vi "Calculate_TargetOffset_Method1.vi"(9 "distance":dbl, 10 "skew":dbl, 11 "depth":dbl) -> (1 "max possible":dbl, 3 "target offset":dbl)   [LabVIEW 2019]
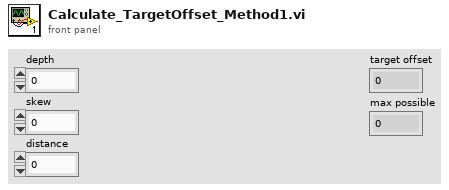
[diagram p1: front panel]
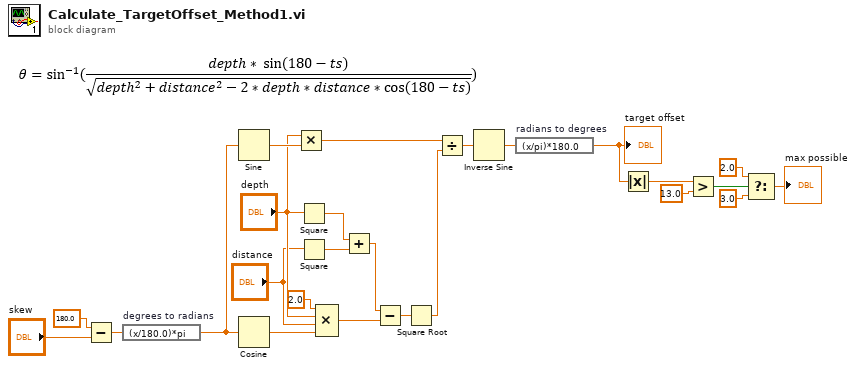
[diagram p0: block diagram]
diagram:
  n1 = Subtract(x=180.0, y="skew") -> (x-y=w23:dbl)
  n2 = expression code="(x/180.0)*pi" "degrees to radians"(w23) -> (w16:dbl)
  n3 = Sine(x=w16) -> (sin(x)=w22:dbl)
  n4 = Cosine(x=w16) -> (cos(x)=w15:dbl)
  n5 = Multiply(x="depth", y=w22) -> (x*y=w11:dbl)
  n6 = Square(x="depth") -> (x^2=w20:dbl)
  n7 = Square(x="distance") -> (x^2=w21:dbl)
  n8 = Compound Arithmetic op=MULTIPLY(2.0 ("value"), "depth", "distance", w15) -> (w13:dbl)
  n9 = Add(x=w20, y=w21) -> (x+y=w14:dbl)
  n10 = Subtract(x=w14, y=w13) -> (x-y=w12:dbl)
  n11 = Square Root(x=w12) -> (sqrt(x)=w10:dbl)
  n12 = Divide(x=w11, y=w10) -> (x/y=w9:dbl)
  n13 = Inverse Sine(1:w9) -> (0:w8:dbl)
  n14 = expression code="(x/pi)*180.0" "radians to degrees"(w8) -> (w7:dbl)
  "target offset" <- w7
  n15 = Absolute Value(x=w7) -> (abs(x)=w6:dbl)
  n16 = Greater?(x=w6, y=13.0) -> (0:w4:bool)
  n17 = Select(t=2.0, s=w4, f=3.0) -> (s? t:f=→"max possible":dbl)
